vi "SMO.UI.Splash.TestLauncher.vi"() -> ()   [LabVIEW 2013, in "SMO.UI.Splash.lvclass"]
doc: "JKI State Machine Objects (SMO) 1.0.0.5\nJKI - JKI\nCopyright (c) 2016, JKI"
uses:
  SMO.UI.Splash.lvclass
  <vilib>/JKI/JKI SMO/SMO/SMO.lvclass
  <vilib>/JKI/JKI SMO/SMO.UI/SMO.UI.lvclass
panel:
  out "error out":errorcluster
  in  "Stop":bool
  # "SMO Splash Test Launcher"
  # "For instructions on how to use the JKI State Machine Objects, examples and video tutorials, visit:\nhttp://jki.net/state-machine-objects/\n\nJKI State Machine Objects™\nhttp://jki.net/state-machine-objects/\nCopyright (C) 2005-2015, JKI <info@jki.net>\nALL RIGHTS RESERVED"
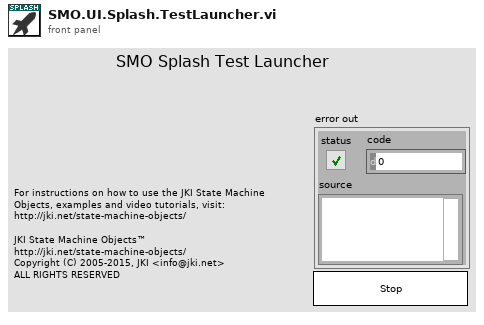
[diagram p1: front panel]
types:
  T1 = cluster{"SMO.UI Public Events":refnum<event-registration>}
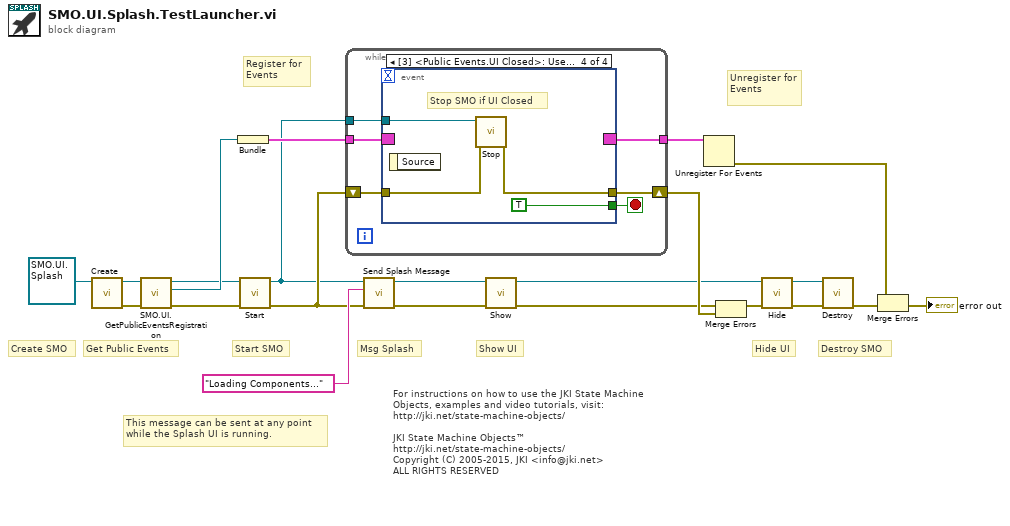
[diagram p0: block diagram]
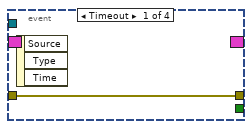
[diagram p2: hidden frame]
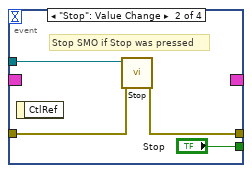
[diagram p3: hidden frame]
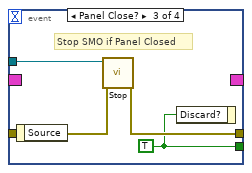
[diagram p4: hidden frame]
diagram:
  # "Msg Splash"
  # "This message can be sent at any point\nwhile the Splash UI is running."
  # "Hide UI"
  # "Show UI"
  # "For instructions on how to use the JKI State Machine Objects, examples and video tutorials, visit:\nhttp://jki.net/state-machine-objects/\n\nJKI State Machine Objects™\nhttp://jki.net/state-machine-objects/\nCopyright (C) 2005-2015, JKI <info@jki.net>\nALL RIGHTS RESERVED"
  # "Get Public Events"
  # "Start SMO"
  # "Destroy SMO"
  # "Create SMO"
  # "Unregister for Events"
  # "Register for Events"
  n1 = call <vilib>:"Create.vi"("SMO"=refnum<class "SMO.UI.Splash.lvclass"> refnum ("SMO.Template.lvclass")) -> ("error out"=w10:errorcluster, "SMO out"=w9:refnum<class "SMO.UI.Splash.lvclass">)  [unwired: 9 in]
  n2 = call <vilib>:"SMO.UI.GetPublicEventsRegistration.vi"("error in (no error)"=w10, "SMO.UI"=w9) -> ("error out"=w5:errorcluster, "SMO.UI Public Events"=w8:refnum<event-registration>, "SMO.UI out"=w6:refnum<class "SMO.UI.Splash.lvclass">)  [unwired: 7 in]
  n3 = Bundle("SMO.UI Public Events"=w8) -> (w21:T1)  [unwired: 1 in]
  n4 = call <vilib>:"Start.vi"("error in (no error)"=w5, "SMO"=w6) -> ("error out"=w4:errorcluster, "SMO out"=w1:refnum<class "SMO.UI.Splash.lvclass">)  [unwired: 8 in]
  n5 = while {
    shift-right: [w27] -> w20
    shift-left: w4 -> [w26]
    tunnel: w21 -> [w25]
    tunnel: [w24] -> w22
    tunnel: w1 -> [w23]
    stop <- w28 stop-if-true
    n6 = event shown="[3] <Public Events.UI Closed>: User Event" {
      selector: w25 -> [_ _ _ _]
      dyn-events: [_ _ _ _] -> w24
      timeout: _ -> [_ _ _ _]
      tunnel: [_ "Stop" w34 TRUE ("OK")] -> w28
      tunnel: w23 -> [_ w31 w37 w41]
      tunnel: [w29 w32 w36 w40] -> w27
      tunnel: w26 -> [w29 w30 w35 w39]
      event Timeout {
        n7 = event-data() -> ()  [unwired: 1 in, 3 out]
      }
      event "Stop": Value Change {
        # "Stop SMO if Stop was pressed"
        n8 = event-data() -> ()  [unwired: 1 in, 1 out]
        n9 = call <vilib>:"Stop.vi"("error in (no error)"=w30, "SMO"=w31) -> ("error out"=w32:errorcluster)  [unwired: 8 in, 1 out]
      }
      event Panel Close? {
        w34 = TRUE ("OK")
        # "Stop SMO if Panel Closed"
        n10 = event-data() -> ()  [unwired: 1 in, 1 out]
        n11 = call <vilib>:"Stop.vi"("error in (no error)"=w35, "SMO"=w37) -> ("error out"=w36:errorcluster)  [unwired: 8 in, 1 out]
        n12 = event-data("Discard?"=w34) -> ()  [unwired: 1 in, 1 out]
      }
      event User Event {
        # "Stop SMO if UI Closed"
        n13 = event-data() -> ()  [unwired: 1 in, 1 out]
        n14 = call <vilib>:"Stop.vi"("error in (no error)"=w39, "SMO"=w41) -> ("error out"=w40:errorcluster)  [unwired: 8 in, 1 out]
      }
    }
  }
  n15 = call-dynamic "Send Splash Message.vi"("error in (no error)"=w4, "Message"="Loading Components...", "SMO.UI.Splash in"=w1) -> ("error out"=w3:errorcluster, "SMO.UI.Splash out"=w2:refnum<class "SMO.UI.Splash.lvclass">)  [unwired: 7 in]
  n16 = call <vilib>:"Show.vi"("error in (no error)"=w3, "SMO.UI"=w2) -> ("error out"=w15:errorcluster, "SMO.UI out"=w14:refnum<class "SMO.UI.Splash.lvclass">)  [unwired: 8 in]
  n17 = Unregister For Events(event registration refnum=w22) -> (error out=w19:errorcluster)  [unwired: 1 in]
  n18 = Merge Errors(w15, w20) -> (w12:errorcluster)
  n19 = call <vilib>:"Hide.vi"("error in (no error)"=w12, "SMO.UI"=w14) -> ("error out"=w11:errorcluster, "SMO.UI out"=w13:refnum<class "SMO.UI.Splash.lvclass">)  [unwired: 8 in]
  n20 = call <vilib>:"Destroy.vi"("error in (no error)"=w11, "SMO"=w13) -> ("error out"=w17:errorcluster)  [unwired: 9 in]
  n21 = Merge Errors(w19, w17) -> (→"error out":errorcluster)
